vi "STAGE+mono+counter_edit24-trial.vi"() -> ()   [LabVIEW 2017]
panel:
  out "Timeout":bool
  out "PROGRESS":sgl(slide) max=10 step=10 scale=0.0..1.0
  in  "?":enum32{"Scan Data", "Scans", "RT Data"}(tab)
  out "Spectrum":cluster{dbl[], dbl[]}(graph)
  out "Decay":cluster{dbl[], dbl[]}[](graph)
  in  "Collect Data!":bool
  out "Waveform Graph":waveform(dbl)[](graph)
  out "?":sgl(knob) scale=0.0..1000000.0
  out "Photon Counts":sgl
  in  "Wavelength":sgl
  in  "Show Real Time Data":bool
  in  "?":enum32{"DELAY", "COUNTER", "MONO", "PLOT"}(tab)
  in  "Data File Path":path
  out "Final time [ps]":sgl
  out "Current time [ps]":sgl
  out "Initial time [ps]":sgl
  in  "Set this as t0":bool
  in  "Axis":u64=1
  in  "Motor ON":bool
  in  "Motor OFF":bool
  out "Current Position [mm]":sgl
  out "Final Position [mm]":sgl
  in  "Data Points":sgl=100.0
  out "Current Point":sgl
  in  "Step Size [um]":sgl=10.0
  in  "Target [mm]":sgl format="%.3f"
  in  "Move":bool
  out "Initial position [mm]":sgl
  in  "GPIB address":string="23"
  in  "Count Mode":sgl(ring) items=["A,B for Preset T", "A-B for Preset T", "A+B for Preset T", "A for Preset B"]
  in  "Trigger mode":u16(ring) items=["10 MHz"=0, "Input 2"=2, "Input T"=3]
  in  "Channel A Input":sgl(ring)=1.0 items=["10 MHz", "Input 1"]
  in  "Channel B Input":u16(ring)=2 items=["Input 1"=1, "Input 2"=2]
  in  "Number of Measurements\n to take at one point/ Number of Periods":sgl=1.0 min=1 max=2000 step=1
  in  "Time between measurements\n at one point (s)/Dwell Time":sgl=0.002 min=0.002 max=60 step=0.001
  in  "gate mode (CW:0)":sgl(slide) scale=0.0..2.0 scale format="%.2f"
  out "Counts":sgl
  in  "Integrating time \nin 10^-7 sec":sgl=10000000.0
  in  "Discriminator Level (mV)":dbl min=-300.0 max=300.0 step=0.2
  in  "Discriminator Slope":bool
  in  "Channel":i16 min=0 max=2 step=1
  out "Current Units \n0=microns\n1=nanometers\n2=angstroms":dbl
  out "Grating #":sgl
  out "Blaze angle":sgl
  out "Grooves/mm":sgl
  out "Mono port":T1(ring)
  out "Time delay":sgl=450000.0 min=1
  in  "Step size":sgl=10.0 min=0
  in  "Scan to":sgl=4000.0
  in  "Scan from":sgl=2600.0
  out "Current wavelength":sgl
  in  "?":bool
  in  "NEW UNIT":T2(ring)
  in  "Array":sgl[](array[numeric])
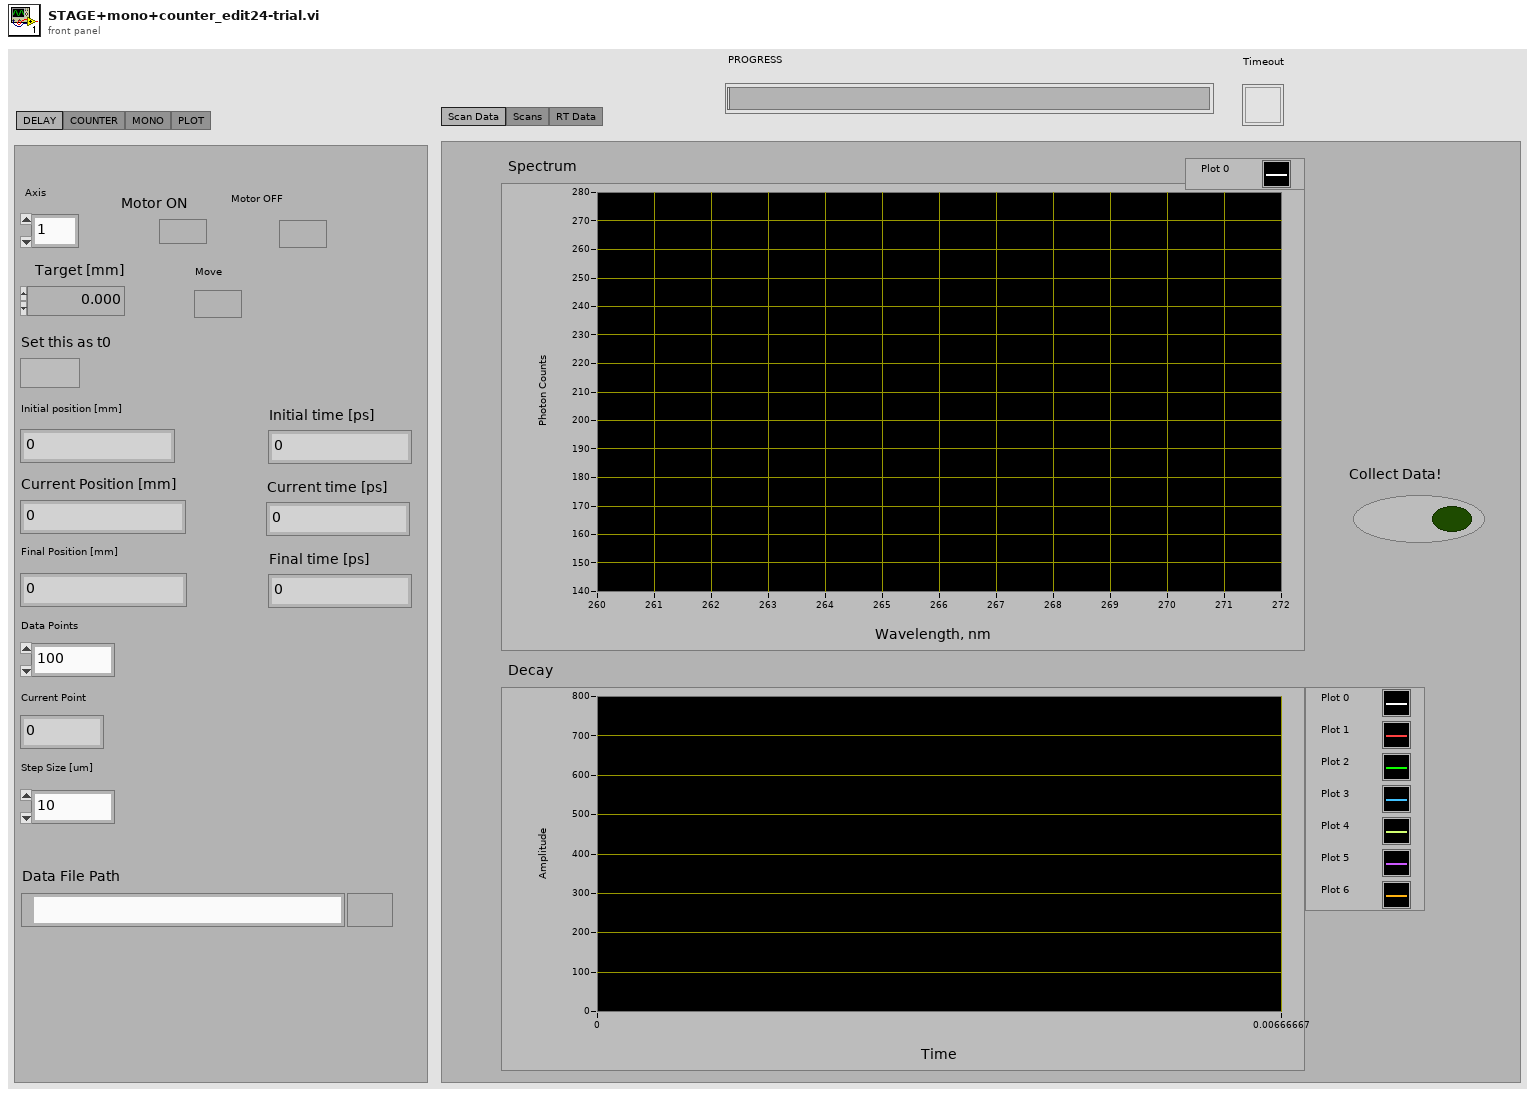
[diagram p1: front panel]
types:
  T1 = enum8{"COM 1", "COM 2", "COM 3", "COM 4", "COM 5", "COM 6", "COM 7", "COM 8", "COM 9"}
  T2 = enum16{"centi-Microns", " Nanometers", "   Angstroms"}
  T3 = cluster{"input XON/XOFF":bool, "input HW Handshake":bool, "input alt HW HShk":bool, "output XON/XOFF":bool, "output HW Handshake":bool, "output alt HW HShk":bool, "XOFF byte":u8, "XON byte":u8, "parity error byte":u16}
  T4 = enum16{"no parity", "odd parity", "even parity", "mark parity", "space parity"}
  T5 = enum16{"open", "replace", "create", "open or create", "replace or create", "replace or create with confirmation"}
  T6 = typedef "NI_Matrix.lvlib/RealMatrix.ctl" = dbl[][]
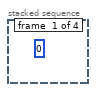
[diagram p2: hidden frame]
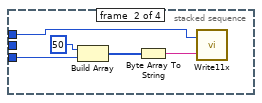
[diagram p3: hidden frame]
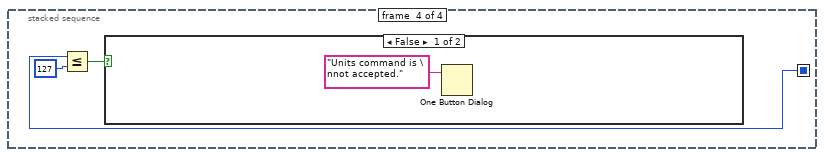
[diagram p4: hidden frame]
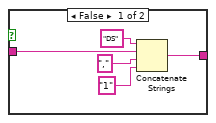
[diagram p7: hidden frame]
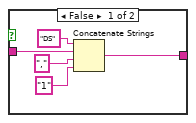
[diagram p9: hidden frame]
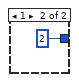
[diagram p13: hidden frame]
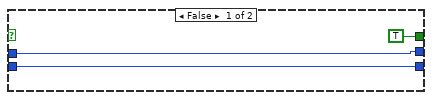
[diagram p14: hidden frame]
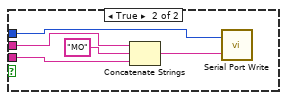
[diagram p15: hidden frame]
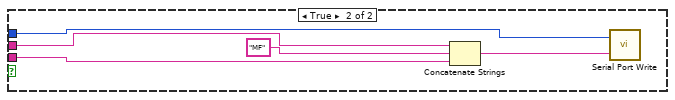
[diagram p16: hidden frame]
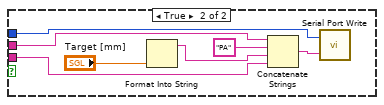
[diagram p17: hidden frame]
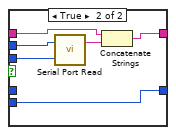
[diagram p19: hidden frame]
diagram:
  w39 = u32 19200  # baud rate
  w38 = u16 8  # data bits
  w37 = enum16{"1 bit", "1.5 bits", "2 bits"}."1 bit"  # stop bits
  w41 = T4."no parity"  # parity
  w19 = 4  # 0=COM1 so n=COM(n+1)
  w40 = u16 1024  # buffer size
  n1 = flat-sequence {
    tunnel: [w44] -> w6
    tunnel: [w43] -> w7
    frame #0 {
      n2 = call "CM Com Read ini.vi"() -> ("Mono port"=w43:T1, "time delay1"=w44:u32)  [unwired: 7 in]
    }
  }
  n3 = call "Query11x.vi"("port number"=w7, "QUERY"=2.0, "time delay"=w6) -> ("STATUS MESSAGE"=→"Grooves/mm":u16)  [unwired: 3 out]
  n4 = call "Query11x.vi"("port number"=w7, "QUERY"=0.0, "time delay"=w6) -> ("STATUS MESSAGE"=→"Current wavelength":u16)  [unwired: 3 out]
  n5 = call "Query11x.vi"("port number"=w7, "QUERY"=14.0, "time delay"=w6) -> ("STATUS MESSAGE"=→"Current Units \n0=microns\n1=nanometers\n2=angstroms":u16)  [unwired: 3 out]
  n6 = call "Query11x.vi"("port number"=w7, "QUERY"=3.0, "time delay"=w6) -> ("STATUS MESSAGE"=→"Blaze angle":u16)  [unwired: 3 out]
  n7 = call "Query11x.vi"("port number"=w7, "QUERY"=14.0, "time delay"=w6) -> ("STATUS MESSAGE"=→"Grating #":u16)  [unwired: 3 out]
  n8 = stacked-sequence {
    seq-local: [_ _ w52 _] -> [_ _ _ w59]
    tunnel: "NEW UNIT" -> [_ w46 _ _]
    tunnel: w7 -> [_ w45 w50 _]
    tunnel: w6 -> [_ _ w51 _]
    frame #0 {
      (unwired) u8 0
    }
    frame #1 {
      n9 = Build Array(u8 50, w46) -> (w48:u16[])
      n10 = Byte Array To String(unsigned byte array=w48) -> (string=w47:string)
      n11 = call "Write11x.vi"("string to write"=w47, "port number"=w45) -> ()  [unwired: 1 out]
    }
    frame #2 {
      n12 = call "Read11x.vi"("response size"=2, "timeout count"=w51, "port number"=w50) -> ("rcv index"=w53:u8[])  [unwired: 2 out]
      n13 = Index Array(array=w53, index=1) -> ()  [unwired: 1 out]
      n14 = Index Array(array=w53, index=0) -> (element=w52:u8)
    }
    frame #3 {
      n15 = Less Or Equal?(x=w59, y=127) -> (x <= y?=w57:bool)
      n16 = case shown="False" w57 {
        frame False {
          n17 = One Button Dialog(message="Units command is \nnot accepted.") -> ()  [unwired: 1 in, 1 out]
        }
        frame True {
        }
      }
    }
  }
  n18 = call "CM Serial Port Setup.vi"("COM port"=w7, "time delay"=w6) -> ("time delay1"=w29:u32, "DK port Out"=w30:T1, "error code"=w32:i32)  [unwired: 7 in]
  n19 = Equal To 0?(x=w32) -> (x = 0?=w31:bool)
  n20 = case shown="True" w31 {
    tunnel: w30 -> [w63 w66]
    tunnel: w29 -> [w62 w65]
    tunnel: [w63 w66] -> w16
    tunnel: [w62 w65] -> w15
    tunnel: [TRUE FALSE] -> w14
    frame False {
    }
    frame True {
      n21 = call "CM Com Write ini.vi"("time delay1"=w66, "Mono port"=w65) -> ()  [unwired: 7 in]
      n22 = local write "Mono port"(w66) -> ()
      n23 = local write "Time delay"(w65) -> ()
    }
  }
  n24 = call <vilib>:"Serial Port Init.vi"("flow control etc."=T3 {"input XON/XOFF"=FALSE, "input HW Handshake"=FALSE, "input alt HW HShk"=FALSE, "output XON/XOFF"=FALSE, "output HW Handshake"=FALSE, "output alt HW HShk"=FALSE, "XOFF byte"=13, "XON byte"=11, "parity error byte"=0}, "parity"=w41, "buffer size"=w40, "stop bits"=w37, "data bits"=w38, "baud rate"=w39, "port number"=w19) -> ("error code"=w36:i32)
  n25 = Concatenate Strings("\r", "\n") -> (w33:string)
  n26 = while {
    tunnel: w15 -> [w69]
    tunnel: w16 -> [w68]
    stop <- TRUE continue-if-true
    n27 = case shown="True" "?" {
      tunnel: w69 -> [_ w72]
      tunnel: w68 -> [_ w71]
      frame False {
      }
      frame True {
        n28 = Two Button Dialog(message="Do you want to change grating?", 1:"No" ("F button name (\"Cancel\")"), 2:"Yes" ("T button name (\"OK\")")) -> (T button?=w73:bool)
        n29 = case shown="True" w73 {
          tunnel: w72 -> [_ w78]
          tunnel: w71 -> [_ w77]
          frame False {
          }
          frame True {
            n30 = Two Button Dialog(message="Disable voltage from PMT", 1:"Do not swich grating" ("F button name (\"Cancel\")"), 2:"Done" ("T button name (\"OK\")")) -> (T button?=w79:bool)
            n31 = case shown="True" w79 {
              tunnel: w78 -> [_ w91]
              tunnel: w77 -> [_ w90]
              frame False {
              }
              frame True {
                n32 = flat-sequence {
                  tunnel: w91 -> [w95]
                  tunnel: [w95] -> w85
                  tunnel: w90 -> [w94]
                  tunnel: [w94] -> w84
                  tunnel: [w92] -> w83
                  tunnel: w85 -> [w100]
                  tunnel: [w100] -> w88
                  tunnel: w84 -> [w101]
                  tunnel: [w101] -> w87
                  tunnel: w83 -> [w99]
                  tunnel: [w99] -> w86
                  tunnel: w88 -> [w105]
                  tunnel: w87 -> [w106]
                  tunnel: [w104] -> w89
                  tunnel: w86 -> [w104]
                  frame #0 {
                    n33 = local read "Grating #"() -> (w93:sgl)
                    n34 = case shown="2, Default" w93 {
                      tunnel: [1 2] -> w92
                      frame 2, Default {
                      }
                      frame 1 {
                      }
                    }
                    n35 = call "Select11x2.vi"("time delay"=w95, "NEW GRT?"=w92, "port number"=w94) -> ()  [unwired: 3 out]
                  }
                  frame #1 {
                    n36 = call "Query11x.vi"("port number"=w101, "QUERY"=u16 2, "time delay"=w100) -> ("STATUS MESSAGE"=w98:u16)  [unwired: 3 out]
                    n37 = local write "Grooves/mm"(w98) -> ()
                  }
                  frame #2 {
                    n38 = Divide(x=w105, y=i16 100 ("device (1)")) -> (x/y=w107:dbl)
                    n39 = call "Query11x.vi"("port number"=w106, "QUERY"=u16 3, "time delay"=w107) -> ("STATUS MESSAGE"=w103:u16)  [unwired: 3 out]
                    n40 = local write "Blaze angle"(w103) -> ()
                  }
                }
                n41 = local write "Grating #"(w89) -> ()
              }
            }
          }
        }
      }
    }
  }
  n42 = while {
    tunnel: w19 -> [w124]
    tunnel: w33 -> [w125]
    tunnel: w36 -> [_]
    tunnel: "Axis" -> [w122]
    stop <- TRUE continue-if-true
    w123 = u32 200  # timeout
    n43 = Format Into String(w122) -> (resulting string=w126:string)  [unwired: 3 in, 1 out]
    n44 = flat-sequence {
      tunnel: w126 -> [w131]
      tunnel: w125 -> [w130]
      tunnel: w124 -> [w132]
      tunnel: w123 -> [w129]
      tunnel: [w131] -> w121
      tunnel: [w130] -> w120
      tunnel: [w132] -> w119
      tunnel: [w129] -> w118
      tunnel: w121 -> [w142]
      tunnel: w120 -> [w141]
      tunnel: w119 -> [w143]
      tunnel: w118 -> [w139]
      tunnel: [w142] -> w117
      tunnel: [w141] -> w116
      tunnel: [w143] -> w115
      tunnel: [w139] -> w114
      tunnel: w117 -> [w152]
      tunnel: w116 -> [w151]
      tunnel: w115 -> [w153]
      tunnel: w114 -> [w149]
      tunnel: [w152] -> w113
      tunnel: [w151] -> w112
      tunnel: [w153] -> w111
      tunnel: [w149] -> w110
      tunnel: w113 -> [w165]
      tunnel: w112 -> [w162]
      tunnel: w111 -> [w164]
      tunnel: w110 -> [w163]
      frame #0 {
        n45 = case shown="False" "Motor ON" {
          tunnel: w132 -> [_ w138]
          tunnel: w131 -> [_ w135]
          tunnel: w130 -> [_ w134]
          frame False {
          }
          frame True {
            n46 = Concatenate Strings(w135, "MO" ("Substring"), w134) -> (w136:string)
            n47 = call <vilib>:"Serial Port Write.vi"("string to write"=w136, "port number"=w138) -> ()  [unwired: 1 out]
          }
        }
      }
      frame #1 {
        n48 = case shown="False" "Motor OFF" {
          tunnel: w143 -> [_ w148]
          tunnel: w142 -> [_ w145]
          tunnel: w141 -> [_ w144]
          frame False {
          }
          frame True {
            n49 = Concatenate Strings(w145, "MF" ("Substring"), w144) -> (w146:string)
            n50 = call <vilib>:"Serial Port Write.vi"("string to write"=w146, "port number"=w148) -> ()  [unwired: 1 out]
          }
        }
      }
      frame #2 {
        n51 = case shown="False" "Move" {
          tunnel: w153 -> [_ w160]
          tunnel: w152 -> [_ w157]
          tunnel: w151 -> [_ w156]
          frame False {
          }
          frame True {
            n52 = Format Into String("Target [mm]") -> (resulting string=w154:string)  [unwired: 3 in, 1 out]
            n53 = Concatenate Strings(w157, "PA" ("Substring"), w154, w156) -> (w158:string)
            n54 = call <vilib>:"Serial Port Write.vi"("string to write"=w158, "port number"=w160) -> ()  [unwired: 1 out]
          }
        }
      }
      frame #3 {
        n55 = case shown="True" "Set this as t0" {
          tunnel: w165 -> [_ w175]
          tunnel: w164 -> [_ w174]
          tunnel: w163 -> [_ w173]
          tunnel: w162 -> [_ w172]
          frame False {
          }
          frame True {
            n56 = flat-sequence {
              tunnel: w175 -> [w179]
              tunnel: w174 -> [w178]
              tunnel: [w178] -> w171
              tunnel: w173 -> [w176]
              tunnel: [w176] -> w170
              tunnel: w172 -> [w177]
              tunnel: w171 -> [w183]
              tunnel: [w183] -> w169
              tunnel: w170 -> [w182]
              tunnel: [w182] -> w168
              tunnel: [w184] -> w167
              tunnel: w169 -> [w189]
              tunnel: w168 -> [w187]
              tunnel: w167 -> [w186]
              tunnel: [w185] -> w166
              tunnel: w166 -> [w211]
              frame #0 {
                # "send position query"
                n57 = Concatenate Strings(w179, "TP" ("Substring"), w177) -> (w180:string)
                n58 = call <vilib>:"Serial Port Write.vi"("string to write"=w180, "port number"=w178) -> ()  [unwired: 1 out]
              }
              frame #1 {
                # "record current time"
                n59 = Tick Count (ms)() -> (millisecond timer value=w184:u32)
              }
              frame #2 {
                # "read characters in serial port"
                n60 = while {
                  shift-left: w186 -> [w190]
                  shift-right: [w191] -> _
                  tunnel: w187 -> [w194]
                  shift-left: "" -> [w197]
                  shift-right: [w196] -> w185
                  tunnel: w189 -> [w198]
                  stop <- w193 continue-if-true
                  n61 = call <vilib>:"Bytes At Serial Port.vi"("port number"=w198) -> ("byte count"=w199:u32)  [unwired: 1 out]
                  n62 = Tick Count (ms)() -> (millisecond timer value=w192:u32)
                  n63 = Subtract(x=w192, y=w190) -> (x-y=w195:u32)
                  n64 = Greater Than 0?(x=w199) -> (x > 0?=w200:bool)
                  n65 = Less?(x=w195, y=w194) -> (x < y?=w193:bool)
                  n66 = case shown="False" w200 {
                    tunnel: w199 -> [_ w208]
                    tunnel: w198 -> [_ w207]
                    tunnel: w197 -> [w202 w205]
                    tunnel: [w202 w204] -> w196
                    tunnel: [w201 w203] -> w191
                    tunnel: w192 -> [_ w203]
                    tunnel: w190 -> [w201 _]
                    frame False {
                    }
                    frame True {
                      n67 = call <vilib>:"Serial Port Read.vi"("requested byte count"=w208, "port number"=w207) -> ("string read"=w206:string)  [unwired: 1 out]
                      n68 = Concatenate Strings(w205, w206) -> (w204:string)
                    }
                  }
                }
              }
              frame #3 {
                n69 = Scan From String(input string=w211) -> (output 1=w209:dbl)  [unwired: 4 in, 3 out]
                n70 = Subtract(x=w209, y=w209) -> (x-y=→"Initial position [mm]":dbl)
              }
            }
          }
        }
      }
    }
    n71 = Wait Until Next ms Multiple(millisecond multiple=u32 50) -> ()  [unwired: 1 out]
  }
  n72 = while {
    tunnel: "GPIB address" -> [w215]
    tunnel: w16 -> [w214]
    tunnel: w15 -> [w213]
    tunnel: w14 -> [w212]
    stop <- TRUE continue-if-true
    n73 = case shown="True" "Show Real Time Data" {
      tunnel: w215 -> [_ w224]
      tunnel: w214 -> [_ w221]
      tunnel: w213 -> [_ w218]
      tunnel: w212 -> [_ w223]
      frame False {
      }
      frame True {
        n74 = flat-sequence {
          tunnel: w224 -> [w253]
          tunnel: "Wavelength" -> [w254]
          tunnel: [w254] -> w235
          tunnel: [w243] -> w234
          tunnel: [w244] -> w233
          tunnel: [w253] -> w232
          tunnel: w218 -> [w244]
          tunnel: w221 -> [w243]
          tunnel: w223 -> [_]
          tunnel: [w242] -> w219
          tunnel: w218 -> [w242]
          tunnel: [w262] -> w231
          tunnel: [w261] -> w230
          tunnel: [w259] -> w229
          tunnel: w235 -> [w257]
          tunnel: w234 -> [w262]
          tunnel: w233 -> [w261]
          tunnel: w232 -> [w259]
          tunnel: [w255] -> w220
          tunnel: w219 -> [w255]
          tunnel: w231 -> [_]
          tunnel: w230 -> [_]
          tunnel: w229 -> [w266]
          tunnel: [w266] -> w228
          tunnel: w221 -> [w265]
          tunnel: w220 -> [w264]
          tunnel: w228 -> [w274]
          tunnel: [w274] -> w227
          tunnel: w227 -> [w324]
          tunnel: [w324] -> w226
          tunnel: w226 -> [w325]
          tunnel: [w325] -> w225
          tunnel: w225 -> [w335]
          frame #0 {
            n75 = call "Query11x.vi"("port number"=w243, "QUERY"=sgl 0.0, "time delay"=w244) -> ("timeout"=w240:bool, "STATUS MESSAGE"=w239:u16)  [unwired: 2 out]
            n76 = call "Query11x.vi"("port number"=w243, "QUERY"=sgl 2.0, "time delay"=w244) -> ("timeout"=w251:bool, "STATUS MESSAGE"=w250:u16)  [unwired: 2 out]
            n77 = call "Query11x.vi"("port number"=w243, "QUERY"=sgl 4.0, "time delay"=w244) -> ("timeout"=w245:bool, "STATUS MESSAGE"=w246:u16)  [unwired: 2 out]
            n78 = call "Query11x.vi"("port number"=w243, "QUERY"=sgl 3.0, "time delay"=w244) -> ("timeout"=w249:bool, "STATUS MESSAGE"=w248:u16)  [unwired: 2 out]
            n79 = local write "Timeout"(w245) -> ()
            n80 = local write "Timeout"(w240) -> ()
            n81 = local write "Timeout"(w251) -> ()
            n82 = local write "Grooves/mm"(w250) -> ()
            n83 = local write "Timeout"(w249) -> ()
            n84 = local write "Blaze angle"(w248) -> ()
            n85 = local write "Grating #"(w246) -> ()
            n86 = Divide(x=w239, y=sgl 10.0 ("Numeric")) -> (x/y=w237:sgl)
            n87 = local write "Current wavelength"(w237) -> ()
          }
          frame #1 {
            n88 = Multiply(x=w257, y=1.0) -> (x*y=w256:dbl)
            n89 = call "Goto11x.vi"("time delay"=w261, "WAVELENGTH"=w256, "port number"=w262) -> ("timeout"=w260:bool)  [unwired: 2 out]
            n90 = local write "Timeout"(w260) -> ()
          }
          frame #2 {
            # "set counter time in 10^-7 seconds in CW"
            n91 = call "Query11x.vi"("port number"=w265, "QUERY"=sgl 0.0, "time delay"=w264) -> ("timeout"=→"Timeout":bool, "STATUS MESSAGE"=w269:u16)  [unwired: 2 out]
            n92 = Divide(x=w269, y=sgl 1.0) -> (x/y=w268:sgl)
            n93 = local write "Current wavelength"(w268) -> ()
          }
          frame #3 {
            # "Configures discriminator."
            n94 = flat-sequence {
              tunnel: w274 -> [w281]
              tunnel: [w281] -> w280
              tunnel: [w288] -> w279
              tunnel: [w286] -> w278
              tunnel: w273 -> [w287]
              tunnel: w280 -> [w286]
              tunnel: w275 -> [w285]
              tunnel: w279 -> [w307]
              tunnel: [w308] -> w277
              tunnel: w278 -> [w306]
              tunnel: [w306] -> w276
              tunnel: w275 -> [w304]
              tunnel: w277 -> [w320]
              tunnel: w276 -> [w319]
              tunnel: w271 -> [w314]
              tunnel: w275 -> [w313]
              frame #0 {
                # "Flush I/O buffers."
                n95 = for {
                  N: sgl 5.0 -> [_]
                  tunnel: w281 -> [w283]
                  n96 = GPIB Write(0:w283, 1:"\r") -> ()  [unwired: 3 in, 2 out]
                }
              }
              frame #1 {
                # "Set discriminator slope."
                n97 = case shown="True" w287 {
                  tunnel: [w294 w299] -> w289
                  tunnel: w285 -> [w293 w298]
                  frame False {
                    n98 = Concatenate Strings("DS", w293, ",", "1") -> (w294:string)
                  }
                  frame True {
                    n99 = Concatenate Strings("DS", w298, ",", "0") -> (w299:string)
                  }
                }
                n100 = GPIB Write(0:w286, 1:w289, 2:sgl 5.0) -> (6:w288:errorcluster)  [unwired: 2 in, 1 out]
              }
              frame #2 {
                # "Set discriminator mode to fixed."
                n101 = Concatenate Strings("DM", w304, ",", "0") -> (w303:string)
                n102 = GPIB Write(0:w306, 1:w303, 2:sgl 5.0, 3:w307) -> (6:w308:errorcluster)  [unwired: 1 in, 1 out]
              }
              frame #3 {
                # "Set discriminator level.\nMust be between +300 and -300 mV."
                n103 = Divide(x=w314, y=1000.0) -> (x/y=w322:dbl)
                n104 = Number To Fractional String(number=w322, precision (6)=sgl 4.0) -> (F-format string=w311:string)  [unwired: 2 in]
                n105 = Concatenate Strings("DL", w313, ",", w311) -> (w318:string)
                n106 = GPIB Write(0:w319, 1:w318, 2:sgl 5.0, 3:w320) -> (6:w315:errorcluster)  [unwired: 1 in, 1 out]
                n107 = call <vilib>:"General Error Handler.vi"("type of dialog (OK msg:1)"=sgl 1.0, "error in (no error)"=w315) -> ()  [unwired: 9 in, 5 out]
              }
            }
            n108 = local read "Discriminator Slope"() -> (w273:bool)
            n109 = local read "Channel"() -> (w272:i16)
            n110 = Number To Decimal String(number=w272) -> (decimal integer string=w275:string)  [unwired: 1 in]
            n111 = local read "Discriminator Level (mV)"() -> (w271:dbl)
          }
          frame #4 {
            n112 = call "Start.vi"("GPIB Address"=w324) -> ()  [unwired: 9 in]
          }
          frame #5 {
            # "Wait for Scan to Finish"
            n113 = for {
              N: sgl 1.0 -> [_]
              tunnel: w325 -> [w327]
              n114 = while {
                tunnel: w327 -> [w328]
                stop <- w330 stop-if-true
                n115 = call "ScanDone.vi"("Wait (ms)"=sgl 1000.0, "GPIB Address"=w328) -> ("Scan Finished?"=w330:bool)
              }
            }
          }
          frame #6 {
            n116 = call "Read Data.vi"("Channel Number"=sgl 0.0, "GPIB Address"=w335, "Number of Datapoints"=sgl 1.0) -> ("Data"=w336:i32[])
            n117 = property class="Knob (strict)"("Scale.Increment"=sgl 1000.0, "Scale.Maximum"=sgl 1000000.0, "Scale.Minimum"=sgl 0.0) -> ()  [unwired: 2 in, 2 out]
            n118 = Index Array(array=w336, index=sgl 0.0) -> (element=→"Photon Counts" →"?":i32)
          }
        }
      }
    }
  }
  n119 = while {
    tunnel: "Axis" -> [w348]
    tunnel: w19 -> [w347]
    tunnel: "GPIB address" -> [w346]
    tunnel: "Integrating time \nin 10^-7 sec" -> [w345]
    tunnel: w15 -> [w344]
    tunnel: w16 -> [w343]
    tunnel: w14 -> [w342]
    stop <- TRUE continue-if-true
    n120 = case shown="True" "Collect Data!" {
      selector: "Collect Data!" -> [_ w349]
      tunnel: w348 -> [_ w357]
      tunnel: w347 -> [_ w356]
      tunnel: w346 -> [_ w355]
      tunnel: w346 -> [_ w353]
      tunnel: w345 -> [_ w352]
      tunnel: w344 -> [_ w351]
      tunnel: w343 -> [_ w354]
      tunnel: w342 -> [_ w350]
      frame False {
      }
      frame True {
        n121 = flat-sequence {
          tunnel: w357 -> [w377]
          tunnel: w356 -> [w375]
          tunnel: w355 -> [w374]
          tunnel: w354 -> [w373]
          tunnel: w353 -> [w372]
          tunnel: w352 -> [w369]
          tunnel: w351 -> [w362]
          tunnel: w350 -> [w361]
          tunnel: w349 -> [_]
          frame #0 {
            w382 = 1000000000000.0
            w387 = sgl 1000.0
            w388 = sgl 300000000.0
            w394 = sgl 1.0
            n122 = Multiply(x="Step Size [um]", y="Data Points") -> (x*y=w391:sgl)
            n123 = Divide(x="Step Size [um]", y=1000.0) -> (x/y=w400:dbl)
            n124 = local read "Initial position [mm]"() -> (w379:sgl)
            n125 = Multiply(x="Scan to", y=w394) -> (x*y=w368:sgl)
            n126 = Increment(x="Data Points") -> (x+1=w409:sgl)
            n127 = Multiply(x="Scan from", y=w394) -> (x*y=w367:sgl)
            n128 = Divide(x=w391, y=sgl 1000.0) -> (x/y=w390:sgl)
            n129 = To Time Stamp(1:w367) -> (0:w397:timestamp)
            n130 = Multiply(x=w368, y=sgl 1.0) -> (x*y=w406:sgl)
            n131 = Multiply(x=sgl 1.0, y=w367) -> (x*y=w371:sgl)
            n132 = Divide(x=w400, y=1000.0) -> (x/y=w401:dbl)
            n133 = for {
              N: w409 -> [_]
              tunnel: w400 -> [w768]
              tunnel: w379 -> [w766]
              tunnel: [w759] -> w408 mode=indexing
              i -> [w767]
              # "distances"
              n134 = Multiply(x=w768, y=w767) -> (x*y=w765:dbl)
              n135 = Add(x=w766, y=w765) -> (x+y=w764:dbl)
              n136 = Divide(x=w764, y=sgl 1000.0) -> (x/y=w758:dbl)
              n137 = Divide(x=w758, y=sgl 300000000.0) -> (x/y=w761:dbl)
              n138 = Multiply(x=w761, y=1000000000000.0) -> (x*y=w759:dbl)
            }
            n139 = Subtract(x=w406, y=w371) -> (x-y=w412:sgl)
            n140 = Divide(x=w379, y=w387) -> (x/y=w385:sgl)
            n141 = Add(x=w379, y=w390) -> (x+y=w381:sgl)
            "Final Position [mm]" <- w381
            n142 = property on="Waveform Graph" class="WFGraph (strict)"("XScale.Increment"="Step size", "XScale.Maximum"=w368, "XScale.Minimum"=w367) -> ()  [unwired: 2 in, 2 out]
            n143 = Divide(x=w381, y=w387) -> (x/y=w386:sgl)
            n144 = Divide(x=w412, y="Step size") -> (x/y=w411:sgl)
            n145 = Divide(x=w385, y=w388) -> (x/y=w384:sgl)
            n146 = Divide(x=w401, y=sgl 300000000.0) -> (x/y=w403:dbl)
            n147 = Bundle By Name("Y"=dbl[] [], "t0"=w397, "dt"="Step size") -> (w396:waveform(dbl))  [unwired: 1 in]
            n148 = Divide(x=w386, y=w388) -> (x/y=w383:sgl)
            n149 = Multiply(x=w403, y=1000000000000.0) -> (x*y=w365:dbl)
            n150 = Multiply(x=w384, y=w382) -> (x*y=w364:dbl)
            "Initial time [ps]" <- w364
            n151 = Round Toward -Infinity(1:w411) -> (0:w370:sgl)
            n152 = Concatenate Strings("\r", "\n") -> (w376:string)
            n153 = Build Array(w396) -> (w360:waveform(dbl)[])
            n154 = Multiply(x=w383, y=w382) -> (x*y=w395:dbl)
            "Final time [ps]" <- w395
            n155 = Increment(x=w370) -> (x+1=w399:sgl)
            n156 = for {
              N: w399 -> [_]
              tunnel: "Step size" -> [w773]
              tunnel: w371 -> [w771]
              tunnel: [w769] -> _ mode=indexing
              i -> [w772]
              # "wavelengths"
              n157 = Multiply(x=w773, y=w772) -> (x*y=w770:sgl)
              n158 = Add(x=w771, y=w770) -> (x+y=w769:sgl)
            }
            n159 = for {
              N: "Data Points" -> [w436]
              tunnel: w379 -> [w477]
              tunnel: "Step Size [um]" -> [w473]
              tunnel: w377 -> [w470]
              tunnel: w376 -> [w467]
              tunnel: w375 -> [w468]
              tunnel: w374 -> [w466]
              tunnel: w373 -> [w464]
              tunnel: w372 -> [w465]
              tunnel: w371 -> [w427]
              tunnel: "Step size" -> [w459]
              tunnel: w370 -> [w458]
              tunnel: w369 -> [w457]
              tunnel: w368 -> [w422]
              tunnel: w367 -> [w421]
              tunnel: "Step size" -> [w423]
              tunnel: w365 -> [w438]
              tunnel: w364 -> [w455]
              shift-right: [w437] -> _
              shift-left: dbl[] [] -> [w433]
              tunnel: w362 -> [w450]
              tunnel: w373 -> [w449]
              tunnel: w361 -> [w448]
              shift-right: [w443] -> _
              shift-left: w360 -> [w444]
              shift-right: [w431] -> _
              shift-left: dbl[][] [] -> [w430]
              shift-right: [w419] -> _
              shift-left: dbl[][] [] -> [w417]
              i -> [w425]
              w447 = dbl[] []
              n160 = stacked-sequence {
                tunnel: w464 -> [w741]
                tunnel: w465 -> [_]
                frame #0 {
                  n161 = call <vilib>:"Close Serial Driver.vi"("port number"=w741) -> ()  [unwired: 1 out]
                  n162 = GPIB Misc(0:"loc 23" ("command string")) -> ()  [unwired: 1 in, 3 out]
                }
              }
              n163 = property on="Waveform Graph" class="WFGraph (strict)"("XScale.Increment"=w423, "XScale.Maximum"=w422, "XScale.Minimum"=w421) -> ()  [unwired: 2 in, 2 out]
              n164 = Number To Decimal String(number=w457) -> (decimal integer string=w462:string)  [unwired: 1 in]
              n165 = Divide(x=w473, y=sgl 1000.0) -> (x/y=w472:sgl)
              n166 = property on="PROGRESS" class="Slide (strict)"("Scale.Increment"=sgl 1.0, "Scale.Maximum"=w436, "Scale.Minimum"=sgl 0.0) -> ()  [unwired: 2 in, 2 out]
              n167 = Multiply(x=w438, y=w425) -> (x*y=w456:dbl)
              n168 = Add(x=sgl 1.0, y=w425) -> (x+y=→"PROGRESS":sgl)
              n169 = Concatenate Strings("CP 2,", w462) -> (w460:string)
              n170 = Add(x=w455, y=w456) -> (x+y=w434:dbl)
              n171 = Multiply(x=w472, y=w425) -> (x*y=w476:sgl)
              n172 = Add(x=w477, y=w476) -> (x+y=w475:sgl)
              n173 = Build Array (concatenate)(w433, w434) -> (w435:dbl[])
              n174 = Format Into String(w470) -> (resulting string=w469:string)  [unwired: 3 in, 1 out]
              n175 = GPIB Write(0:w466, 1:w460, 2:sgl 5.0 ("mode (0)")) -> ()  [unwired: 2 in, 2 out]
              n176 = flat-sequence {
                tunnel: w475 -> [w744]
                tunnel: [w744] -> w471
                tunnel: w467 -> [w746]
                tunnel: w469 -> [w745]
                tunnel: w468 -> [w742]
                tunnel: w471 -> [w755]
                tunnel: [w750] -> w420
                frame #0 {
                  n177 = Format Into String(w744) -> (resulting string=w743:string)  [unwired: 3 in, 1 out]
                  n178 = Wait (ms)(milliseconds to wait=sgl 100.0) -> ()  [unwired: 1 out]
                  n179 = Concatenate Strings(w745, "PA" ("Substring"), w743, w746) -> (w748:string)
                  n180 = call <vilib>:"Serial Port Write.vi"("string to write"=w748, "port number"=w742) -> ()  [unwired: 1 out]
                }
                frame #1 {
                  n181 = Divide(x=w755, y=sgl 1000.0) -> (x/y=w753:sgl)
                  n182 = Wait (ms)(milliseconds to wait=sgl 1000.0) -> ()  [unwired: 1 out]
                  n183 = Divide(x=w753, y=sgl 300000000.0) -> (x/y=w752:sgl)
                  n184 = Multiply(x=w752, y=1000000000000.0) -> (x*y=w750:dbl)
                  "Current time [ps]" <- w750
                  "Current Position [mm]" <- w755
                }
              }
              n185 = Add(x=w425, y=sgl 1.0) -> (x+y=w424:sgl)
              n186 = flat-sequence {
                tunnel: w466 -> [w503]
                tunnel: w427 -> [w502]
                tunnel: w459 -> [w501]
                tunnel: w458 -> [w500]
                tunnel: w422 -> [w499]
                tunnel: w421 -> [w498]
                tunnel: w447 -> [w497]
                tunnel: w447 -> [w496]
                tunnel: w423 -> [w495]
                tunnel: w450 -> [w494]
                tunnel: w449 -> [w493]
                tunnel: w448 -> [w492]
                tunnel: [w490] -> w446
                tunnel: [w491] -> _
                tunnel: [w490] -> w445
                tunnel: w424 -> [w489]
                tunnel: w420 -> [w488]
                tunnel: [w487] -> w418
                tunnel: w417 -> [w486]
                tunnel: w446 -> [w719]
                tunnel: [w722] -> w432
                tunnel: [w721] -> w429
                tunnel: [w720] -> w419
                tunnel: w418 -> [w720]
                frame #0 {
                  # "step size"
                  n187 = while {
                    tunnel: w503 -> [w545]
                    tunnel: w502 -> [w566]
                    tunnel: w501 -> [w538]
                    tunnel: w500 -> [w565]
                    tunnel: w499 -> [w541]
                    tunnel: w498 -> [w540]
                    tunnel: w495 -> [w542]
                    shift-right: [w562] -> w490
                    shift-left: w496 -> [w561]
                    shift-right: [w557] -> w491
                    shift-left: w497 -> [w564]
                    tunnel: w494 -> [w505]
                    tunnel: w493 -> [w504]
                    tunnel: w492 -> [w547]
                    tunnel: w489 -> [w526]
                    tunnel: w488 -> [w514]
                    shift-right: [w507] -> w487
                    shift-left: w486 -> [w506]
                    i -> [w534]
                    stop <- w536 stop-if-true
                    n188 = property on="Spectrum" class="XYGraph (strict)"("XScale.Increment"=w542, "XScale.Maximum"=w541, "XScale.Minimum"=w540) -> ()  [unwired: 2 in, 2 out]
                    n189 = Multiply(x=sgl 1.0, y=w538) -> (x*y=w537:sgl)
                    n190 = Multiply(x=w534, y=w537) -> (x*y=w567:sgl)
                    n191 = Greater Or Equal?(x=w534, y=w565) -> (x >= y?=w536:bool)
                    n192 = Add(x=w567, y=w566) -> (x+y=w546:sgl)
                    n193 = Add(x=w534, y=sgl 1.0) -> (x+y=w527:sgl)
                    n194 = Build Array (concatenate)(w564, w546) -> (w563:dbl[])
                    n195 = flat-sequence {
                      tunnel: w545 -> [w578]
                      tunnel: w546 -> [w579]
                      tunnel: [w579] -> w551
                      tunnel: [w569] -> w550
                      tunnel: [w570] -> w549
                      tunnel: [w578] -> w548
                      tunnel: w505 -> [w570]
                      tunnel: w504 -> [w569]
                      tunnel: w547 -> [_]
                      tunnel: [w577] -> w528
                      tunnel: w527 -> [w577]
                      tunnel: [w576] -> w515
                      tunnel: w514 -> [w576]
                      tunnel: w506 -> [w575]
                      tunnel: [w575] -> w513
                      tunnel: [w589] -> w556
                      tunnel: [w588] -> w555
                      tunnel: [w586] -> w554
                      tunnel: w551 -> [w582]
                      tunnel: w550 -> [w589]
                      tunnel: w549 -> [w588]
                      tunnel: w548 -> [w586]
                      tunnel: [w583] -> w529
                      tunnel: w528 -> [w583]
                      tunnel: [w582] -> w521
                      tunnel: [w581] -> w516
                      tunnel: w515 -> [w581]
                      tunnel: w513 -> [w580]
                      tunnel: [w580] -> w512
                      tunnel: w556 -> [_]
                      tunnel: w555 -> [_]
                      tunnel: w554 -> [w599]
                      tunnel: [w599] -> w544
                      tunnel: [w598] -> w530
                      tunnel: w529 -> [w598]
                      tunnel: [w597] -> w522
                      tunnel: w521 -> [w597]
                      tunnel: [w596] -> w517
                      tunnel: w516 -> [w596]
                      tunnel: w512 -> [w595]
                      tunnel: [w595] -> w511
                      tunnel: w504 -> [w594]
                      tunnel: w505 -> [w592]
                      tunnel: w504 -> [w593]
                      tunnel: w544 -> [w609]
                      tunnel: [w609] -> w543
                      tunnel: [w608] -> w531
                      tunnel: w530 -> [w608]
                      tunnel: [w607] -> w523
                      tunnel: w522 -> [w607]
                      tunnel: [w606] -> w518
                      tunnel: w517 -> [w606]
                      tunnel: w511 -> [w605]
                      tunnel: [w605] -> w510
                      tunnel: w543 -> [w666]
                      tunnel: [w666] -> w553
                      tunnel: [w665] -> w532
                      tunnel: w531 -> [w665]
                      tunnel: [w664] -> w524
                      tunnel: w523 -> [w664]
                      tunnel: [w663] -> w519
                      tunnel: w518 -> [w663]
                      tunnel: w510 -> [w662]
                      tunnel: [w662] -> w509
                      tunnel: w553 -> [w671]
                      tunnel: [w671] -> w552
                      tunnel: [w670] -> w533
                      tunnel: w532 -> [w670]
                      tunnel: [w669] -> w525
                      tunnel: w524 -> [w669]
                      tunnel: [w668] -> w520
                      tunnel: w519 -> [w668]
                      tunnel: w509 -> [w667]
                      tunnel: [w667] -> w508
                      tunnel: [w682] -> w559
                      tunnel: w552 -> [w714]
                      tunnel: w533 -> [w680]
                      tunnel: w526 -> [w683]
                      tunnel: w525 -> [w684]
                      tunnel: w520 -> [w686]
                      tunnel: w508 -> [w681]
                      tunnel: [w679] -> w507
                      frame #0 {
                        n196 = call "Query11x.vi"("port number"=w569, "QUERY"=sgl 0.0, "time delay"=w570) -> ("timeout"=w573:bool, "STATUS MESSAGE"=w572:u16)  [unwired: 2 out]
                        n197 = local write "Timeout"(w573) -> ()
                        n198 = Divide(x=w572, y=1 ("Numeric")) -> (x/y=w568:dbl)
                        n199 = local write "Current wavelength"(w568) -> ()
                      }
                      frame #1 {
                        n200 = Multiply(x=w582, y=sgl 1.0) -> (x*y=w584:sgl)
                        n201 = call "Goto11x.vi"("time delay"=w588, "WAVELENGTH"=w584, "port number"=w589) -> ("timeout"=w587:bool)  [unwired: 2 out]
                        n202 = local write "Timeout"(w587) -> ()
                      }
                      frame #2 {
                        # "set counter time in 10^-7 seconds in CW"
                        n203 = call "Query11x.vi"("port number"=w594, "QUERY"=sgl 0.0, "time delay"=w592) -> ("timeout"=w603:bool, "STATUS MESSAGE"=w602:u16)  [unwired: 2 out]
                        n204 = call "Query11x.vi"("port number"=w593, "QUERY"=14.0, "time delay"=w592) -> ("STATUS MESSAGE"=w590:u16)  [unwired: 3 out]
                        n205 = local write "Timeout"(w603) -> ()
                        n206 = local write "Current Units \n0=microns\n1=nanometers\n2=angstroms"(w590) -> ()
                        n207 = Divide(x=w602, y=sgl 1.0) -> (x/y=w601:sgl)
                        n208 = local write "Current wavelength"(w601) -> ()
                      }
                      frame #3 {
                        # "Configures discriminator."
                        n209 = flat-sequence {
                          tunnel: w609 -> [w619]
                          tunnel: [w619] -> w618
                          tunnel: [w626] -> w617
                          tunnel: [w624] -> w616
                          tunnel: "Discriminator Slope" -> [w625]
                          tunnel: w618 -> [w624]
                          tunnel: w610 -> [w623]
                          tunnel: w617 -> [w645]
                          tunnel: [w646] -> w615
                          tunnel: w616 -> [w644]
                          tunnel: [w644] -> w614
                          tunnel: w610 -> [w642]
                          tunnel: w615 -> [w658]
                          tunnel: w614 -> [w657]
                          tunnel: "Discriminator Level (mV)" -> [w652]
                          tunnel: w610 -> [w651]
                          frame #0 {
                            # "Flush I/O buffers."
                            n210 = for {
                              N: sgl 5.0 -> [_]
                              tunnel: w619 -> [w621]
                              n211 = GPIB Write(0:w621, 1:"\r") -> ()  [unwired: 3 in, 2 out]
                            }
                          }
                          frame #1 {
                            # "Set discriminator slope."
                            n212 = case shown="True" w625 {
                              tunnel: [w632 w637] -> w627
                              tunnel: w623 -> [w631 w636]
                              frame False {
                                n213 = Concatenate Strings("DS", w631, ",", "1") -> (w632:string)
                              }
                              frame True {
                                n214 = Concatenate Strings("DS", w636, ",", "0") -> (w637:string)
                              }
                            }
                            n215 = GPIB Write(0:w624, 1:w627, 2:sgl 5.0) -> (6:w626:errorcluster)  [unwired: 2 in, 1 out]
                          }
                          frame #2 {
                            # "Set discriminator mode to fixed."
                            n216 = Concatenate Strings("DM", w642, ",", "0") -> (w641:string)
                            n217 = GPIB Write(0:w644, 1:w641, 2:sgl 5.0, 3:w645) -> (6:w646:errorcluster)  [unwired: 1 in, 1 out]
                          }
                          frame #3 {
                            # "Set discriminator level.\nMust be between +300 and -300 mV."
                            n218 = Divide(x=w652, y=1000.0) -> (x/y=w660:dbl)
                            n219 = Number To Fractional String(number=w660, precision (6)=sgl 4.0) -> (F-format string=w649:string)  [unwired: 2 in]
                            n220 = Concatenate Strings("DL", w651, ",", w649) -> (w656:string)
                            n221 = GPIB Write(0:w657, 1:w656, 2:sgl 5.0, 3:w658) -> (6:w653:errorcluster)  [unwired: 1 in, 1 out]
                            n222 = call <vilib>:"General Error Handler.vi"("type of dialog (OK msg:1)"=1, "error in (no error)"=w653) -> ()  [unwired: 9 in, 5 out]
                          }
                        }
                        n223 = Number To Decimal String(number="Channel") -> (decimal integer string=w610:string)  [unwired: 1 in]
                      }
                      frame #4 {
                        n224 = call "Start.vi"("GPIB Address"=w666) -> ()  [unwired: 9 in]
                      }
                      frame #5 {
                        # "Wait for Scan to Finish"
                        n225 = for {
                          N: sgl 1.0 -> [_]
                          tunnel: w671 -> [w673]
                          n226 = while {
                            tunnel: w673 -> [w674]
                            stop <- w676 stop-if-true
                            n227 = call "ScanDone.vi"("Wait (ms)"=1000, "GPIB Address"=w674) -> ("Scan Finished?"=w676:bool)
                          }
                        }
                      }
                      frame #6 {
                        w685 = sgl 0.0
                        w693 = "\r\n"
                        n228 = call "Read Data.vi"("Channel Number"=sgl 0.0, "GPIB Address"=w714, "Number of Datapoints"=sgl 1.0) -> ("Data"=w715:i32[])
                        n229 = Index Array(array=w715, index=sgl 0.0) -> (element=w682:i32)
                        "Counts" <- w682
                        n230 = local read "Integrating time \nin 10^-7 sec"() -> (w691:sgl)
                        n231 = Replace Array Subset(array=w681, new element #1=w682, index (row) #1=w680, index (col) #1=w683, new element #2=w684, index (row) #2=w680, index (col) #2=w685, new element #3=w686, index (row) #3=w685, index (col) #3=w683) -> (w679:T6)
                        n232 = Array To Spreadsheet String(delimiter (Tab)=",", array=w679, 3:"%f" ("format string")) -> (spreadsheet string=w692:string)
                        n233 = local read "Blaze angle"() -> (w709:sgl)
                        n234 = local read "Grating #"() -> (w708:sgl)
                        n235 = Multiply(x=w691, y=1e-07) -> (x*y=w690:dbl)
                        n236 = Get Date/Time In Seconds() -> (seconds since 1Jan1904=w703:timestamp)
                        n237 = Format Date/Time String(time format string (%c)="%Y-%b-%d %H:%M:%S", seconds (now)=w703) -> (date/time string=w704:string)  [unwired: 1 in]
                        n238 = Number To Decimal String(number=w690) -> (decimal integer string=w705:string)  [unwired: 1 in]
                        n239 = Number To Decimal String(number=w708) -> (decimal integer string=w706:string)  [unwired: 1 in]
                        n240 = Number To Decimal String(number=w709) -> (decimal integer string=w694:string)  [unwired: 1 in]
                        n241 = call <vilib>:"Space Constant.vi"() -> ("String"=w707:string)
                        n242 = Open/Create/Replace File(file path (use dialog)="Data File Path", operation (0:open)=T5."replace or create") -> (refnum out=w713:refnum<file>)  [unwired: 4 in, 2 out]
                        n243 = Concatenate Strings(w693, "Data was taken on ", w704, w693, "Integration Time is ", w705, w707, "s", w693, "Monochromator gratng # ", w706, "; ", "blazed for ", w694, w707, "nm", w693, w693, w693, w692) -> (w688:string)
                        n244 = Write to Text File(file (use dialog)=w713, text=w688) -> (refnum out=w678:refnum<file>)  [unwired: 2 in, 2 out]
                        n245 = Flush File(refnum=w678) -> (refnum out=w677:refnum<file>)  [unwired: 1 in, 1 out]
                        n246 = Close File(refnum=w677) -> ()  [unwired: 1 in, 2 out]
                      }
                    }
                    n247 = Build Array (concatenate)(w561, w559) -> (w560:dbl[])
                    n248 = Bundle(w563, w560) -> (w558:cluster{dbl[], dbl[]})  [unwired: 1 in]
                    "Spectrum" <- w558
                    n249 = Unbundle(w558) -> (w557:dbl[], w562:dbl[])
                  }
                }
                frame #1 {
                  n250 = Array Size(array="Array") -> (size(s)=w721:i32)
                  n251 = flat-sequence {
                    tunnel: w719 -> [w728]
                    tunnel: "Array" -> [w727]
                    tunnel: w721 -> [w726]
                    tunnel: [w724] -> w722
                    frame #0 {
                      n252 = for {
                        N: w726 -> [_]
                        tunnel: w727 -> [w739]
                        tunnel: w728 -> [w734]
                        shift-right: [w729] -> w724
                        shift-left: dbl[] [] -> [w730]
                        i -> [w732]
                        n253 = local read "Scan from"() -> (w737:sgl)
                        n254 = Index Array(array=w739, index=w732) -> (element=w738:sgl)
                        n255 = local read "Step size"() -> (w735:sgl)
                        n256 = Subtract(x=w738, y=w737) -> (x-y=w736:sgl)
                        n257 = Divide(x=w736, y=w735) -> (x/y=w733:sgl)
                        n258 = Index Array(array=w734, index=w733) -> (element=w731:dbl)
                        n259 = Insert Into Array(array=w730, index=w732, new element=w731) -> (w729:dbl[])
                      }
                    }
                  }
                }
              }
              n260 = local read "Scan from"() -> (w441:sgl)
              n261 = local read "Step size"() -> (w439:sgl)
              n262 = To Time Stamp(1:w441) -> (0:w440:timestamp)
              n263 = Bundle By Name("Y"=w445, "t0"=w440, "dt"=w439) -> (w442:waveform(dbl))  [unwired: 1 in]
              n264 = Build Array (concatenate)(w444, w442) -> (w443:waveform(dbl)[])
              "Waveform Graph" <- w443
              n265 = for {
                N: w429 -> [_]
                tunnel: [w485] -> w437
                tunnel: w435 -> [w484]
                tunnel: w432 -> [w482]
                tunnel: [w481] -> w431
                tunnel: w430 -> [w483]
                tunnel: [w478] -> w428 mode=indexing
                i -> [w480]
                n266 = Build Array (concatenate)(w483, w482) -> (w481:dbl[][])
                n267 = Index Array(array=w482, index=w480) -> ()  [unwired: 1 out]
                n268 = Index Array(array=w481, index (col)=w480) -> (element=w479:dbl[])  [unwired: 1 in]
                n269 = Bundle(w484, w479) -> (w478:cluster{dbl[], dbl[]})  [unwired: 1 in]
                n270 = Unbundle(w478) -> (w485:dbl[])  [unwired: 1 out]
              }
              "Decay" <- w428
              "Current Point" <- w425
            }
            n271 = property on="Decay" class="XYGraph (strict)"("XScale.Increment"=w365, "XScale.Maximum"=w395, "XScale.Minimum"=w364) -> ()  [unwired: 2 in, 2 out]
            n272 = Build Array (concatenate)(sgl 0.0, w408) -> ()  [unwired: 1 out]
          }
        }
      }
    }
  }
  n273 = call "Configure.vi"("Dwell Time (s)"="Time between measurements\n at one point (s)/Dwell Time", "Channel T Input"="Trigger mode", "Channel B Input"="Channel B Input", "Channel A Input"="Channel A Input", "Integrating time, 10^-7 sec"="Integrating time \nin 10^-7 sec", "gate mode (CW:0)"="gate mode (CW:0)", "Scan End Mode"=FALSE, "Number of Periods"="Number of Measurements\n to take at one point/ Number of Periods", "Count Mode"="Count Mode", "GPIB Address"="GPIB address") -> ()
  "Mono port" <- w7
  "Time delay" <- w6
